vi "RangeI2C-single.vi"(0 "Remote IP Address":string="192.168.124.53", 1 "Remote Port":u16=502, 2 "I2C Operation Control":T1(ring)=enum."Command Find Range", 3 "SCL DIO Ch. No.":u16=2, 4 "SDA DIO Ch. No.":u16=3, 5 "CURRENT 8-bit address (dec.)":u16=200, 8 "NEW 8-bit address (dec.)":u8=224) -> (6 "Range (cm)":dbl=27.0, 7 "Range (in.)":dbl=10.62992125984252)   [LabVIEW 2022 SP3]
panel:
  in  "stop":bool
  # "Even address values up to 254\n\nInvalid Address Values: 0, 80, 164, 170"
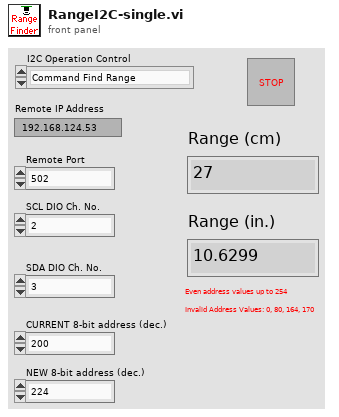
[diagram p1: front panel]
types:
  T1 = enum16{"Configure I2C Settings", "Command Find Range", "Command Read Range", "Report the last range value", "Change sensor address", "Wait to range 100ms"}
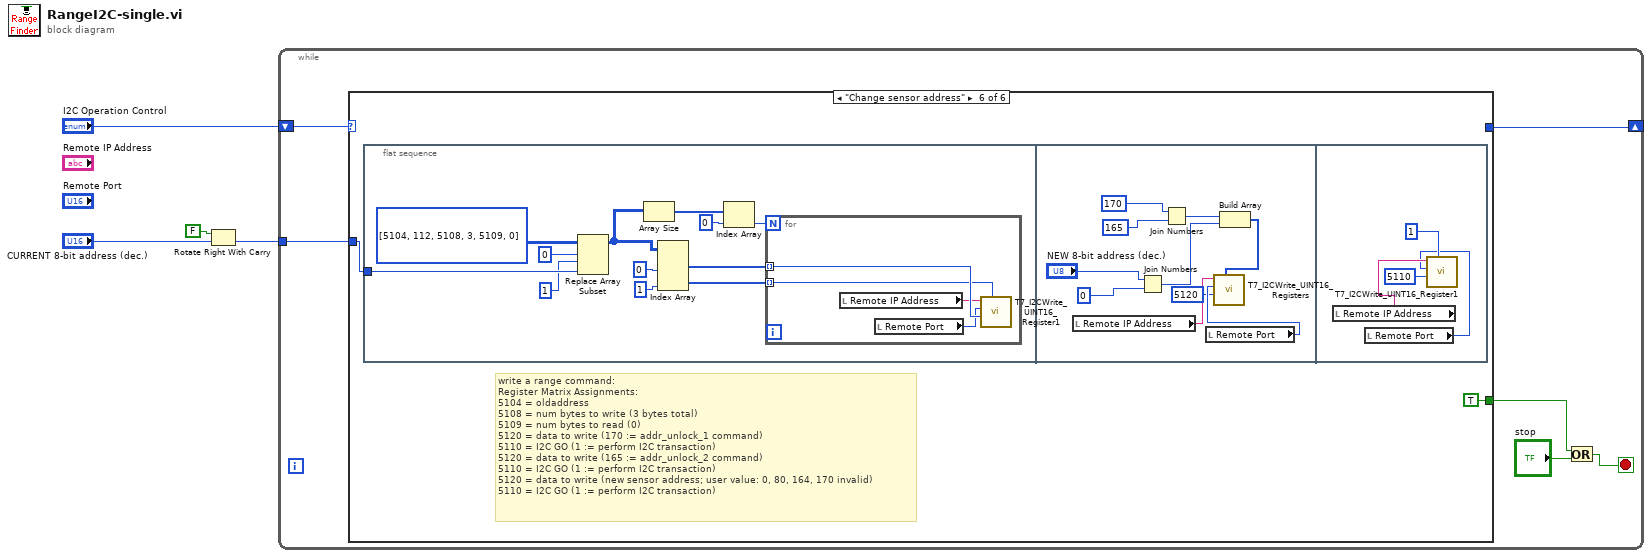
[diagram p0: block diagram]
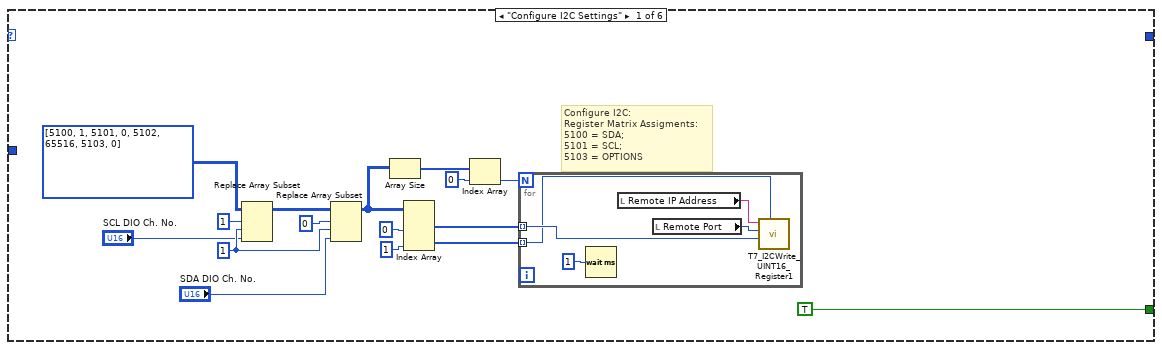
[diagram p2: hidden frame]
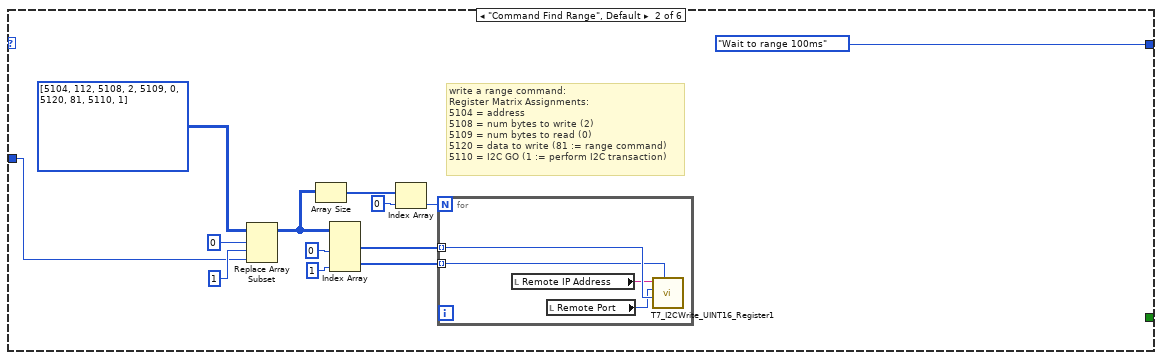
[diagram p3: hidden frame]
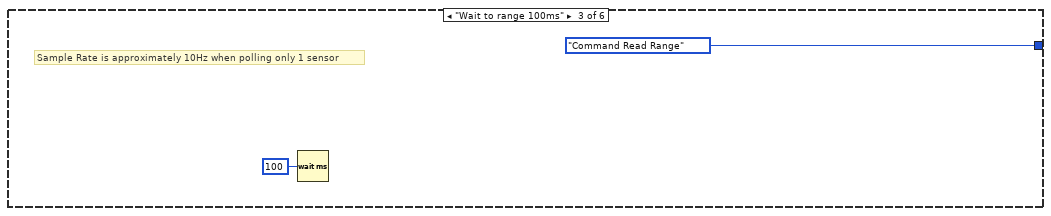
[diagram p4: hidden frame]
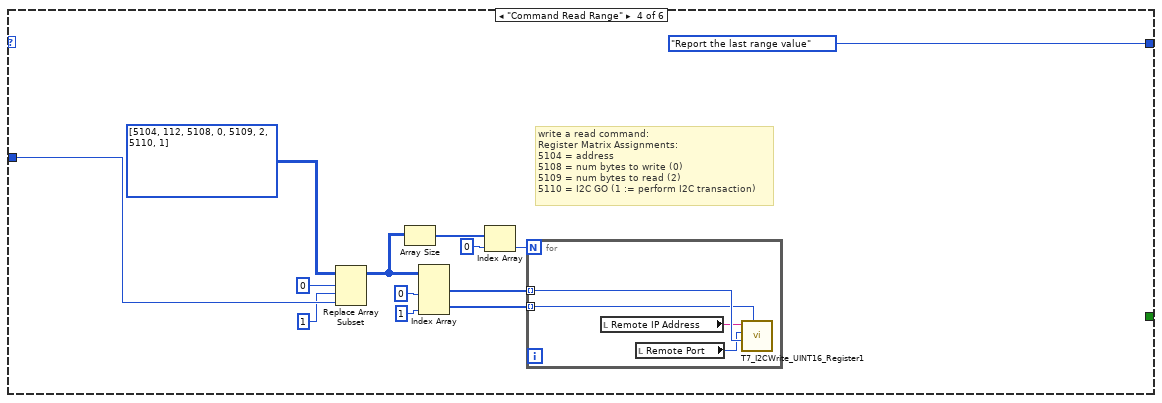
[diagram p5: hidden frame]
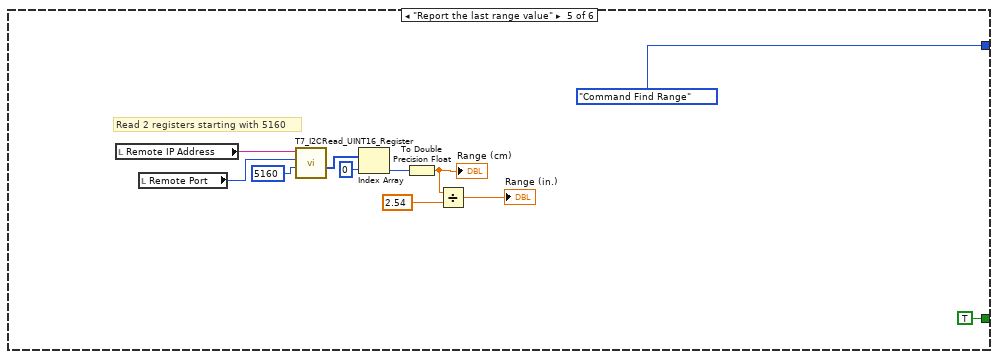
[diagram p6: hidden frame]
diagram:
  n1 = Rotate Right With Carry(2:"CURRENT 8-bit address (dec.)", 3:FALSE ("carry")) -> (0:w1:u16)  [unwired: 1 out]
  n2 = while {
    tunnel: w1 -> [w10]
    shift-right: [w9] -> _
    shift-left: "I2C Operation Control" -> [w5]
    stop <- w6 stop-if-true
    n3 = case shown="\"Change sensor address\"" w5 {
      tunnel: w10 -> [_ w34 _ w63 _ w80]
      tunnel: [_ T1."Wait to range 100ms" ("I2C Operation Control") T1."Command Read Range" ("I2C Operation Control") T1."Report the last range value" ("I2C Operation Control") T1."Command Find Range" ("I2C Operation Control") _] -> w9
      tunnel: [TRUE ("x") _ _ _ TRUE ("x") TRUE ("x")] -> w7
      frame "Configure I2C Settings" {
        w16 = 1 ("disabled index (col)")
        # "Configure I2C: \nRegister Matrix Assigments:\n5100 = SDA;\n5101 = SCL;\n5103 = OPTIONS"
        n4 = Replace Array Subset(array=i32[][] [[5100, 1], [5101, 0], [5102, 65516], [5103, 0]], new element="SCL DIO Ch. No.", index (row)=1, index (col)=w16) -> (w15:i32[][])
        n5 = Replace Array Subset(array=w15, new element="SDA DIO Ch. No.", index (row)=0, index (col)=w16) -> (w12:i32[][])
        n6 = Array Size(array=w12) -> (size(s)=w26:i32[])
        n7 = Index Array(array=w12, index (col) #1=0 ("disabled index (col)"), index (col) #2=1 ("index (col)")) -> (element #1=w21:i32[], element #2=w20:i32[])  [unwired: 2 in]
        n8 = Index Array(array=w26, index=0) -> (element=w24:i32)
        n9 = for {
          N: w24 -> [_]
          tunnel: w21 -> [w31] mode=indexing
          tunnel: w20 -> [w30] mode=indexing
          n10 = Wait (ms)(milliseconds to wait=u32 1) -> ()  [unwired: 1 out]
          n11 = local read "Remote IP Address"() -> (w29:string)
          n12 = local read "Remote Port"() -> (w28:u16)
          n13 = call "T7_I2CWrite_UINT16_Register1.vi"("Remote IP Address"=w29, "Remote Port"=w28, "Starting Address"=w31, "UINT16 to Write"=w30) -> ()  [unwired: 5 in, 2 out]
        }
      }
      frame "Command Find Range", Default {
        # "write a range command:\nRegister Matrix Assignments:\n5104 = address\n5108 = num bytes to write (2)\n5109 = num bytes to read (0)\n5120 = data to write (81 := range command)\n5110 = I2C GO (1 := perform I2C transaction)"
        n14 = Replace Array Subset(array=i32[][] [[5104, 112], [5108, 2], [5109, 0], [5120, 81], [5110, 1]], new element=w34, index (row)=0, index (col)=1 ("disabled index (col)")) -> (w33:i32[][])
        n15 = Array Size(array=w33) -> (size(s)=w44:i32[])
        n16 = Index Array(array=w33, index (col) #1=0 ("disabled index (col)"), index (col) #2=1 ("index (col)")) -> (element #1=w39:i32[], element #2=w38:i32[])  [unwired: 2 in]
        n17 = Index Array(array=w44, index=0) -> (element=w42:i32)
        n18 = for {
          N: w42 -> [_]
          tunnel: w39 -> [w48] mode=indexing
          tunnel: w38 -> [w47] mode=indexing
          n19 = local read "Remote IP Address"() -> (w46:string)
          n20 = local read "Remote Port"() -> (w45:u16)
          n21 = call "T7_I2CWrite_UINT16_Register1.vi"("Remote IP Address"=w46, "Remote Port"=w45, "Starting Address"=w48, "UINT16 to Write"=w47) -> ()  [unwired: 5 in, 2 out]
        }
      }
      frame "Wait to range 100ms" {
        # "Sample Rate is approximately 10Hz when polling only 1 sensor"
        n22 = Wait (ms)(milliseconds to wait=u32 100) -> ()  [unwired: 1 out]
      }
      frame "Command Read Range" {
        # "write a read command:\nRegister Matrix Assignments:\n5104 = address\n5108 = num bytes to write (0)\n5109 = num bytes to read (2)\n5110 = I2C GO (1 := perform I2C transaction)"
        n23 = Replace Array Subset(array=i32[][] [[5104, 112], [5108, 0], [5109, 2], [5110, 1]], new element=w63, index (row)=0, index (col)=1 ("disabled index (col)")) -> (w51:i32[][])
        n24 = Array Size(array=w51) -> (size(s)=w52:i32[])
        n25 = Index Array(array=w51, index (col) #1=0 ("disabled index (col)"), index (col) #2=1 ("index (col)")) -> (element #1=w57:i32[], element #2=w58:i32[])  [unwired: 2 in]
        n26 = Index Array(array=w52, index=0) -> (element=w54:i32)
        n27 = for {
          N: w54 -> [_]
          tunnel: w57 -> [w67] mode=indexing
          tunnel: w58 -> [w66] mode=indexing
          n28 = local read "Remote IP Address"() -> (w65:string)
          n29 = local read "Remote Port"() -> (w64:u16)
          n30 = call "T7_I2CWrite_UINT16_Register1.vi"("Remote IP Address"=w65, "Remote Port"=w64, "Starting Address"=w67, "UINT16 to Write"=w66) -> ()  [unwired: 5 in, 2 out]
        }
      }
      frame "Report the last range value" {
        # "Read 2 registers starting with 5160"
        n31 = local read "Remote IP Address"() -> (w76:string)
        n32 = local read "Remote Port"() -> (w77:u16)
        n33 = call "T7_I2CRead_UINT16_Register.vi"("FirstChannel"=5160, "Remote Port"=w77, "Remote IP Address"=w76) -> ("Raw Data Read"=w75:u16[])  [unwired: 6 in, 2 out]
        n34 = Index Array(array=w75, index=0) -> (element=w73:u16)
        n35 = To Double Precision Float(number=w73) -> (double precision float=w69:dbl)
        "Range (cm)" <- w69
        n36 = Divide(x=w69, y=2.54) -> (x/y=→"Range (in.)":dbl)
      }
      frame "Change sensor address" {
        # "write a range command:\nRegister Matrix Assignments:\n5104 = oldaddress\n5108 = num bytes to write (3 bytes total)\n5109 = num bytes to read (0)\n5120 = data to write (170 := addr_unlock_1 command)\n5110 = I2C GO (1 := perform I2C transaction)\n5120 = data to write (165 := addr_unlock_2 command)\n5110 = I2C GO (1 := perform I2C transaction)\n5120 = data to write (new sensor address; user value: 0, 80, 164, 170 invalid)\n5110 = I2C GO (1 := perform I2C transaction)"
        n37 = flat-sequence {
          tunnel: w80 -> [w83]
          frame #0 {
            n38 = Replace Array Subset(array=i32[][] [[5104, 112], [5108, 3], [5109, 0]], new element=w83, index (row)=0, index (col)=1 ("disabled index (col)")) -> (w81:i32[][])
            n39 = Array Size(array=w81) -> (size(s)=w92:i32[])
            n40 = Index Array(array=w81, index (col) #1=0 ("disabled index (col)"), index (col) #2=1 ("index (col)")) -> (element #1=w87:i32[], element #2=w86:i32[])  [unwired: 2 in]
            n41 = Index Array(array=w92, index=0) -> (element=w90:i32)
            n42 = for {
              N: w90 -> [_]
              tunnel: w87 -> [w96] mode=indexing
              tunnel: w86 -> [w95] mode=indexing
              n43 = local read "Remote IP Address"() -> (w94:string)
              n44 = local read "Remote Port"() -> (w93:u16)
              n45 = call "T7_I2CWrite_UINT16_Register1.vi"("Remote IP Address"=w94, "Remote Port"=w93, "Starting Address"=w96, "UINT16 to Write"=w95) -> ()  [unwired: 5 in, 2 out]
            }
          }
          frame #1 {
            n46 = local read "Remote IP Address"() -> (w99:string)
            n47 = Join Numbers(hi="NEW 8-bit address (dec.)", lo=u8 0) -> ((hi.lo)=w101:u16)
            n48 = Join Numbers(hi=u8 170, lo=u8 165) -> ((hi.lo)=w102:u16)
            n49 = local read "Remote Port"() -> (w98:u16)
            n50 = Build Array(w102, w101) -> (w100:u16[])
            n51 = call "T7_I2CWrite_UINT16_Registers.vi"("Remote IP Address"=w99, "Remote Port"=w98, "Starting Address"=u16 5120, "UINT16 to Write"=w100) -> ()  [unwired: 5 in, 2 out]
          }
          frame #2 {
            n52 = local read "Remote IP Address"() -> (w108:string)
            n53 = local read "Remote Port"() -> (w107:u16)
            n54 = call "T7_I2CWrite_UINT16_Register1.vi"("Remote IP Address"=w108, "Remote Port"=w107, "Starting Address"=u16 5110, "UINT16 to Write"=u16 1) -> ()  [unwired: 5 in, 2 out]
          }
        }
      }
    }
    n55 = Or(x=w7, y="stop") -> (x .or. y?=w6:bool)
  }
